vi "AnalogOutputCommand.vi"(6 "AnalogOutputCommand":cluster{"Name":string, "Value":u16}, 7 "msg in":string) -> (3 "msg out":string)   [LabVIEW 2016]
doc: "Flattens an analog output command into a message"
uses:
  std_msgs/subs/stringScalar.vi
  std_msgs/subs/u16Scalar.vi
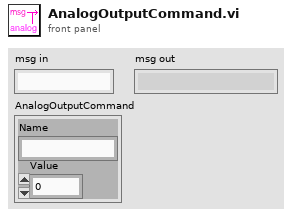
[diagram p1: front panel]
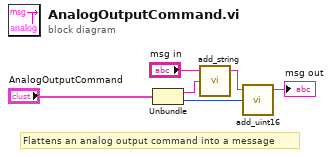
[diagram p0: block diagram]
diagram:
  # "Flattens an analog output command into a message"
  n1 = Unbundle("AnalogOutputCommand") -> ("Name"=w5:string, "Value"=w3:u16)
  n2 = call-poly "add_string.vi"("String"=w5, "msg in"="msg in") -> ("msg out"=w2:string)  [unwired: 3 in]
  n3 = call-poly "add_uint16.vi"("Numeric"=w3, "msg in"=w2) -> ("msg out"=→"msg out":string)  [unwired: 3 in]
